vi "Add Label.vi"(6 "transfer type":T2, 8 "error in":errorcluster, 9 "SDI value":T3=-1 items=["All"=-1, "0 (b00)"=0, "1 (b01)"=1, "2 (b10)"=2, "3 (b11)"=3], 10 "label value":u32, 11 "port ref":T1 format="%.0x") -> (0 "error out":errorcluster, 2 "label ref":T1 format="%.0x", 3 "port ref out":T1 format="%.0x")   [LabVIEW 2020, in "ARINC 429 Scripting.lvlib"]
uses:
  ARINC 429 Scripting.lvlib
  Shared/SDI.ctl
  Shared/Transfer Type.ctl
  <vilib>/NI VeriStand/Custom Device API/Custom Device Item Ref.ctl
  Shared/Label Properties.ctl
  <vilib>/NI VeriStand/Custom Device API/Custom Device Channel.ctl
  <vilib>/NI VeriStand/Custom Device API/Custom Device Channel Type.ctl
  Ballard/Constants.vi
  <vilib>/NI VeriStand/Custom Device API/Set Item Property (U16).vi
  Ballard/Ballard ARINC 429 Scripting.lvlib
  <vilib>/NI VeriStand/Custom Device API/Custom Device API.lvlib
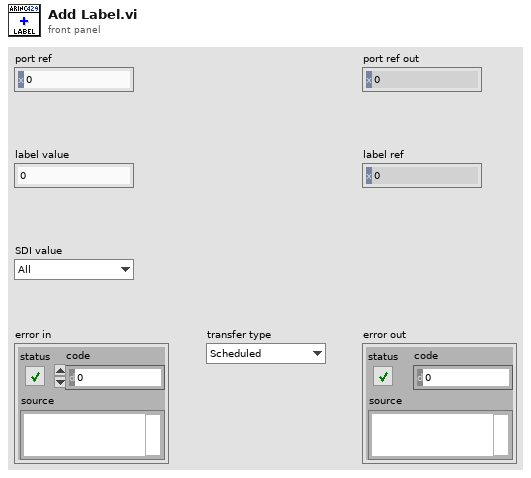
[diagram p1: front panel]
types:
  T1 = typedef "Custom Device API.lvlib/Custom Device Item Ref.ctl" = u64
  T2 = typedef "Transfer Type.ctl" = enum16{"Scheduled", "Acyclic", "Block", "Strobe"}
  T3 = typedef "SDI.ctl" = i32
  T4 = typedef "Label Properties.ctl" = cluster{"label (Dec)":u32, "SDI value":u8, "SDI enabled":bool}
  T5 = typedef "Direction.ctl" = enum16{"Rx", "Tx"}
  T6 = typedef "Custom Device API.lvlib/Custom Device Channel.ctl" = cluster{"Type":T7, "Units":string, "Default Value":dbl, "Faultable":bool, "Scalable":bool}
  T7 = typedef "Custom Device API.lvlib/Custom Device Channel Type.ctl" = enum16{"Input", "Output"}
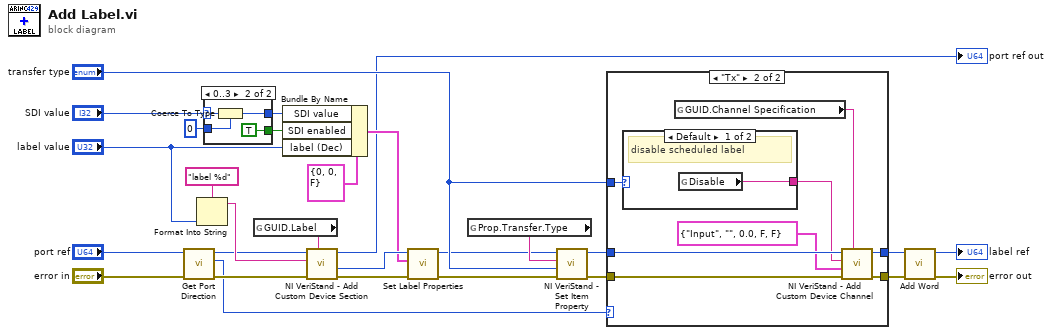
[diagram p0: block diagram]
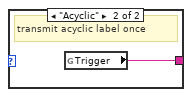
[diagram p4: hidden frame]
diagram:
  n1 = call "Get Port Direction.vi"("error in"="error in", "port ref in"="port ref") -> ("error out"=w8:errorcluster, "direction"=w7:T5, "port ref out"=w9:T1)  [unwired: 7 in]
  n2 = Format Into String(format string="label %d", "label value") -> (resulting string=w16:string)  [unwired: 2 in, 1 out]
  n3 = case shown="0..3" "SDI value" {
    selector: "SDI value" -> [_ w32]
    tunnel: [w29 w33] -> w5
    tunnel: u8 0 ("SDI value") -> [w29 w31]
    tunnel: [_ TRUE] -> w3
    frame Default {
    }
    frame 0..3 {
      n4 = Coerce To Type(0:w32, 1:w31) -> (2:w33:u8)
    }
  }
  n5 = global read "Constants.vi" "GUID.Label"() -> (w17:string)
  n6 = Bundle By Name(cluster=T4 {"label (Dec)"=0, "SDI value"=0, "SDI enabled"=FALSE} ("label properties"), "SDI value"=w5, "SDI enabled"=w3, "label (Dec)"="label value") -> (w13:T4)
  n7 = call <vilib>:"NI VeriStand - Add Custom Device Section.vi"("GUID (Default Section)"=w17, "error in (no error)"=w8, "Section Name"=w16, "Parent Ref in"=w9) -> ("error out"=w19:errorcluster, "Section Ptr"=w18:T1, "Parent Ref out"=→"port ref out":T1)  [unwired: 4 in, 1 out]
  n8 = call "Set Label Properties.vi"("error in"=w19, "label properties"=w13, "label ref"=w18) -> ("error out"=w21:errorcluster, "label ref out"=w20:T1)  [unwired: 7 in]
  n9 = global read "Constants.vi" "Prop.Transfer.Type"() -> (w22:string)
  n10 = call-poly <vilib>:"NI VeriStand - Set Item Property.vi"("error in (no error)"=w21, "Value"="transfer type", "Property Name"=w22, "Item Ref in"=w20) -> ("error out"=w23:errorcluster, "Item Ref out"=w25:T1)  [unwired: 5 in, 1 out]
  n11 = case shown="\"Tx\"" w7 {
    tunnel: w23 -> [w34 w43]
    tunnel: [w34 w42] -> w24
    tunnel: w25 -> [w35 w41]
    tunnel: [w35 w40] -> w26
    tunnel: "transfer type" -> [_ w38]
    frame "Rx", Default {
    }
    frame "Tx" {
      n12 = case shown="Default" w38 {
        tunnel: [w44 w45] -> w37
        frame Default {
          # "disable scheduled label"
          n13 = global read "Constants.vi" "Disable"() -> (w44:string)
        }
        frame "Acyclic" {
          # "transmit acyclic label once"
          n14 = global read "Constants.vi" "Trigger"() -> (w45:string)
        }
      }
      n15 = global read "Constants.vi" "GUID.Channel Specification"() -> (w39:string)
      n16 = call <vilib>:"NI VeriStand - Add Custom Device Channel.vi"("GUID (Default Channel)"=w39, "error in (no error)"=w43, "Channel"=T6 {"Type"=enum."Input", "Units"="", "Default Value"=0.0, "Faultable"=FALSE, "Scalable"=FALSE}, "Channel Name"=w37, "Parent Ref in"=w41) -> ("error out"=w42:errorcluster, "Parent Ref out"=w40:T1)  [unwired: 3 in, 2 out]
    }
  }
  n17 = call "Add Word.vi"("error in"=w24, "label ref"=w26) -> ("error out"=→"error out":errorcluster, "label ref out"=→"label ref":T1)  [unwired: 6 in, 2 out]
